vi "filter_images_by_xi.vi"(8 "Error In":errorcluster, 10 "Xi":T1, 11 "Image Names":string[](array[string])) -> (0 "Error Out":errorcluster, 3 "Filtered Image Names":string[](array[string]))   [LabVIEW 2019]
uses:
  xi_angles_enum_typedef.ctl
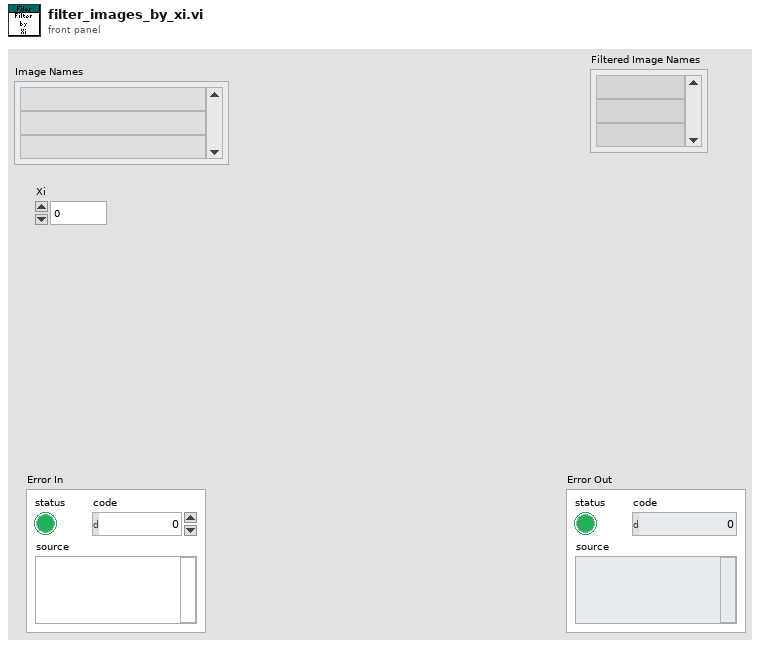
[diagram p1: front panel]
types:
  T1 = typedef "xi_angles_enum_typedef.ctl" = enum16{"0", "45"}
  T2 = typedef "image_property_cluster_typedef.ctl" = cluster{"Stage Angle":dbl, "Sample Angle":dbl, "Polarizer 1 Angle":dbl, "Polarizer 2 Angle":dbl, "Sample Name":string}
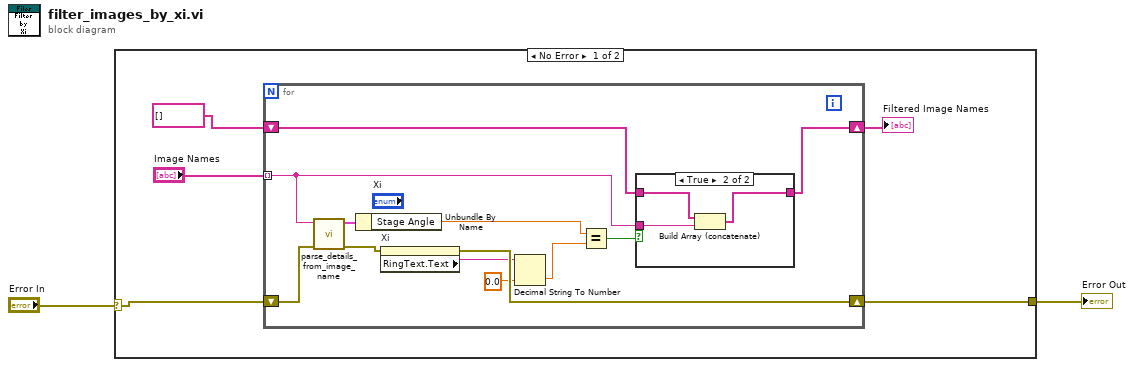
[diagram p0: block diagram]
diagram:
  n1 = case shown="No Error" "Error In" {
    selector: "Error In" -> [w6 w24]
    tunnel: [w5 w24] -> w1
    frame No Error {
      n2 = for {
        tunnel: "Image Names" -> [w9] mode=indexing
        shift-right: [w16] -> w5
        shift-left: w6 -> [w15]
        shift-right: [w8] -> w3
        shift-left: string[] [] -> [w10]
        n3 = call "parse_details_from_image_name.vi"("Error In"=w15, "Image Name"=w9) -> ("Error Out"=w17:errorcluster, "Image Properties"=w19:T2)  [unwired: 8 in]
        n4 = Unbundle By Name(w19) -> ("Stage Angle"=w18:dbl)
        n5 = property on="Xi" class="Enum (strict)"(error in=w17) -> (error out=w16:errorcluster, "RingText.Text"=w14:string)  [unwired: 1 in, 1 out]
        n6 = Decimal String To Number(string=w14, default (0L)=0.0) -> (number=w12:dbl)  [unwired: 1 in, 1 out]
        n7 = Equal?(x=w18, y=w12) -> (x = y?=w11:bool)
        n8 = case shown="True" w11 {
          tunnel: w10 -> [w20 w23]
          tunnel: w9 -> [_ w22]
          tunnel: [w20 w21] -> w8
          frame False {
          }
          frame True {
            n9 = Build Array (concatenate)(w23, w22) -> (w21:string[])
          }
        }
      }
      "Filtered Image Names" <- w3
    }
    frame Error {
    }
  }
  "Error Out" <- w1
